vi "Main.vi"(11 "Module Admin":refnum<class "Delacor_lib_QMH_Module Admin.lvclass">) -> ()   [LabVIEW 2020, in "Dinero.lvlib"]
doc: "This template is based off of the Queued Message Handler design pattern and the Queued Message Handler project template that ships with LabVIEW.\n\nThe main difference is that the queue is private to this module and communication between modules is performed via Broadcast and Request events.\n\nRequest events are wrapped in public API methods and are handled in the Event Handling Loop (EHL) of this VI. Any module can register for Broadcast events sent by this module. The EHL generates messages based on user interface actions.\n\nThe Message Handling Loop (MHL) processes messages generated by the EHL, or by other messages. The messages are string values, so new messages can be added easily to the Message Cases case structure in the MHL. Each message cluster can also provide an optional value for Message Data, which is a variant that can be converted to whatever message-specific data is required.\n_____\nBased on DQMH Project Template 6.0.0.91."
uses:
  Dinero.lvlib
  <vilib>/Delacor/Delacor QMH/Libraries/Module Admin_class/Delacor_lib_QMH_Module Admin.lvclass
  Module Data--cluster.ctl
  Stop Argument--cluster.ctl
  <vilib>/Delacor/Delacor QMH/Libraries/Message Queue_class/Delacor_lib_QMH_Message Queue.lvclass/Delacor_lib_QMH_Message Queue.ctl
  <vilib>/Delacor/Delacor QMH/Libraries/Module Admin_class/Delacor_lib_QMH_Module Admin.lvclass/Delacor_lib_QMH_Module Admin.ctl
  DRAW FP IN UI Argument--cluster.ctl
  Moneda 1 Argument--cluster.ctl
  Moneda 2 Argument--cluster.ctl
  Moneda 5 Argument--cluster.ctl
  Moneda 10 Argument--cluster.ctl
  <vilib>/Utility/miscctls.llb/LVPointTypeDef.ctl
  <vilib>/Delacor/Delacor QMH/Libraries/Message Queue_class/Delacor_lib_QMH_Enqueue Message (Single).vi
  <vilib>/Delacor/Delacor QMH/Libraries/Module Admin_class/Delacor_lib_QMH_Get External Launch.vi
  <vilib>/Utility/error.llb/Error Cluster From Error Code.vi
  <vilib>/ErrorRing/Error Ring.xnode
  <vilib>/Delacor/Delacor QMH/Libraries/Message Queue_class/Delacor_lib_QMH_Message Queue.lvclass
panel:
  out "Cambio":i32
  out "Credito":i32
  in  "Moneda 4":bool
  in  "Moneda 3":bool
  in  "Moneda 2":bool
  in  "Moneda 1":bool
  out "error out":errorcluster
  out "Status":string
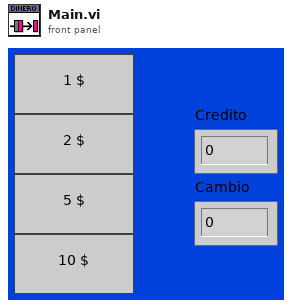
[diagram p1: front panel]
types:
  T1 = typedef "Dinero.lvlib/Request Events--cluster.ctl" = cluster{"Stop Module":refnum<user-event>, "Show Panel":refnum<user-event>, "Hide Panel":refnum<user-event>, "Get Module Execution Status":refnum<user-event>, "Show Diagram":refnum<user-event>, "DRAW FP IN UI":refnum<user-event>, "Moneda 1":refnum<user-event>, "Moneda 2":refnum<user-event>, "Moneda 5":refnum<user-event>, "Moneda 10":refnum<user-event>}
  T2 = typedef "Dinero.lvlib/Module Data--cluster.ctl" = cluster{"Status":string, "Credito":i32, "Cambio":i32}
  T3 = enum32{"invalid lock state", "Not Locked", "Locked (No Password)", "Password-protected"}
  T4 = typedef "Dinero.lvlib/Stop Argument--cluster.ctl" = cluster{"Origin":string, "Exit via Stop Module Req?":bool, "Wait for Module to stop?":bool}
  T5 = typedef "Dinero.lvlib/DRAW FP IN UI Argument--cluster.ctl" = cluster{"Sub Panel Dinero":refnum<vi>}
  T6 = typedef "Dinero.lvlib/Moneda 1 Argument--cluster.ctl" = cluster{"Boolean":bool}
  T7 = typedef "Dinero.lvlib/Moneda 2 Argument--cluster.ctl" = cluster{"Boolean":bool}
  T8 = typedef "Dinero.lvlib/Moneda 5 Argument--cluster.ctl" = cluster{"Boolean":bool}
  T9 = typedef "Dinero.lvlib/Moneda 10 Argument--cluster.ctl" = cluster{"Boolean":bool}
  T10 = typedef "LVPointTypeDef.ctl" = cluster{"Horizontal":i16, "Vertical":i16}
  T11 = enum32{"Invalid", "Standard", "Closed", "Hidden", "Minimized", "Maximized"}
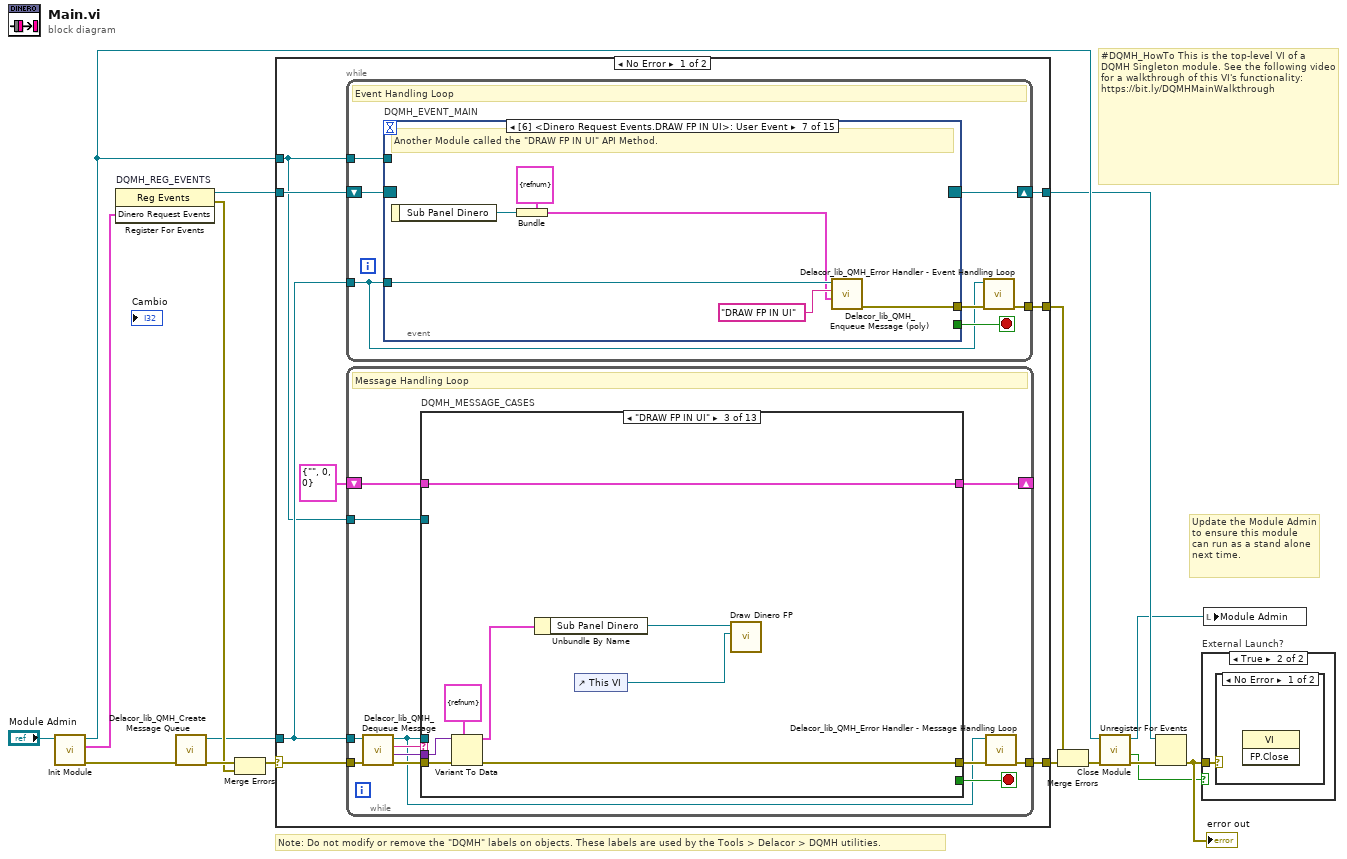
[diagram p0: block diagram]
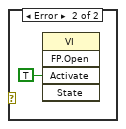
[diagram p3: hidden frame]
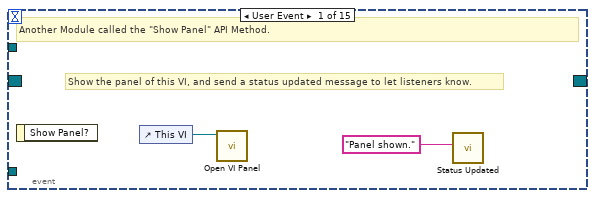
[diagram p4: hidden frame]
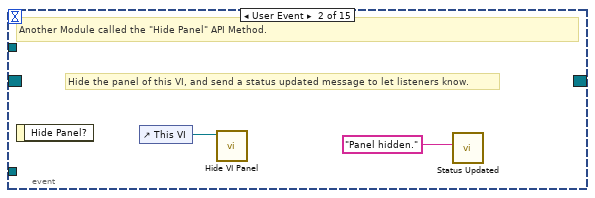
[diagram p5: hidden frame]
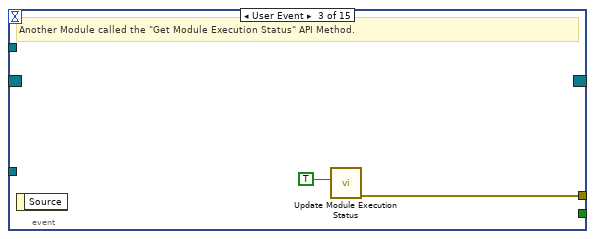
[diagram p6: hidden frame]
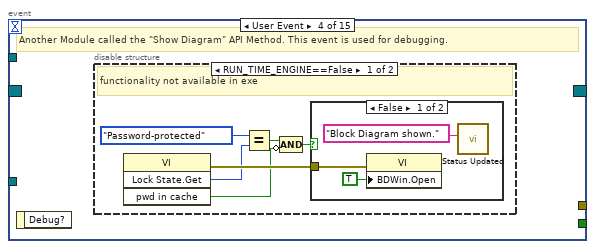
[diagram p7: hidden frame]
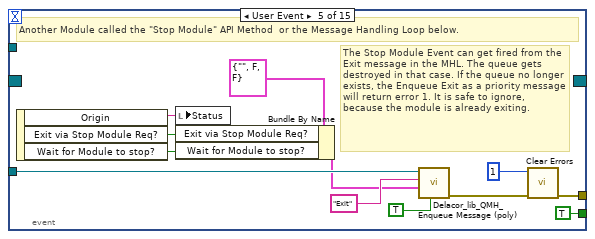
[diagram p10: hidden frame]
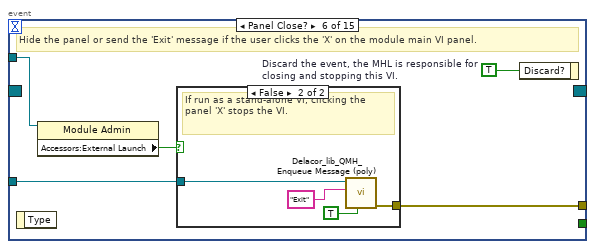
[diagram p11: hidden frame]
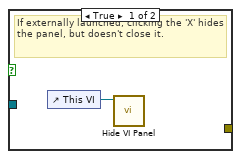
[diagram p12: hidden frame]
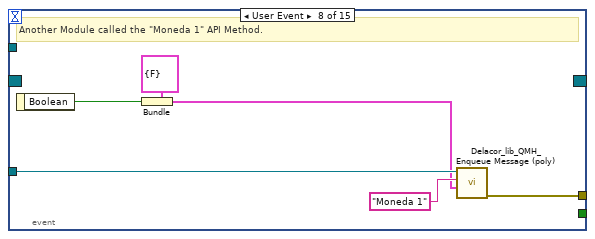
[diagram p13: hidden frame]
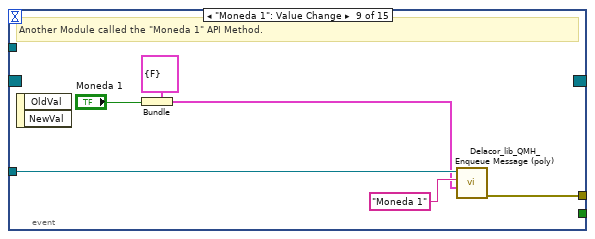
[diagram p14: hidden frame]
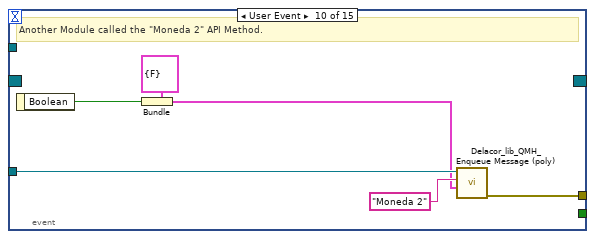
[diagram p15: hidden frame]
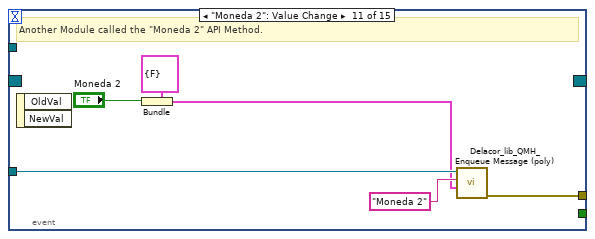
[diagram p16: hidden frame]
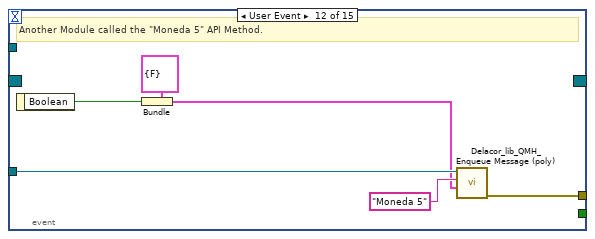
[diagram p17: hidden frame]
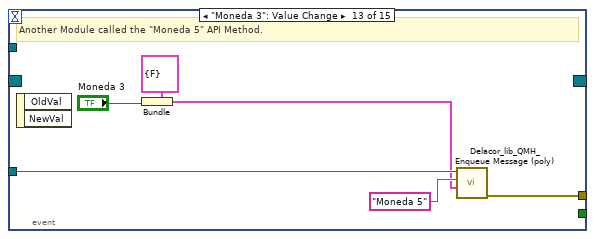
[diagram p18: hidden frame]
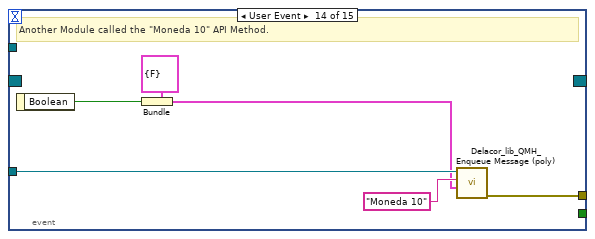
[diagram p19: hidden frame]
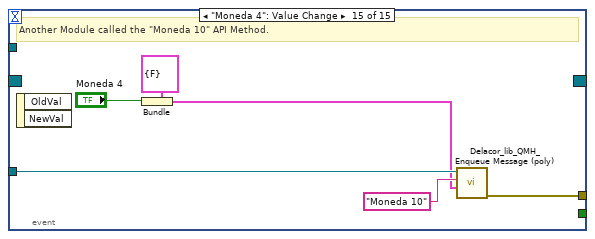
[diagram p20: hidden frame]
diagram:
  # "#DQMH_HowTo This is the top-level VI of a DQMH Singleton module. See the following video for a walkthrough of this VI's functionality: https://bit.ly/DQMHMainWalkthrough"
  # "Note: Do not modify or remove the \"DQMH\" labels on objects. These labels are used by the Tools > Delacor > DQMH utilities."
  # "Update the Module Admin to ensure this module can run as a stand alone next time."
  n1 = call "Init Module.vi"("Singleton Module Admin in"="Module Admin") -> ("error out"=w16:errorcluster, "Dinero Request Events"=w5:T1, "Singleton Module Admin out"=w8:refnum<class "Delacor_lib_QMH_Module Admin.lvclass">)  [unwired: 8 in]
  n2 = register-events "DQMH_REG_EVENTS"(w5) -> (reference out=w6:refnum<event-registration>, error out=w9:errorcluster)  [unwired: 2 in]
  n3 = call <vilib>:"Delacor_lib_QMH_Create Message Queue.vi"("error in"=w16) -> ("error out"=w11:errorcluster, "Message Queue"=w4:refnum<class "Delacor_lib_QMH_Message Queue.lvclass">)  [unwired: 9 in]
  n4 = Merge Errors(w11, w9) -> (w10:errorcluster)
  n5 = case shown="No Error" w10 {
    selector: w10 -> [w23 w273]
    tunnel: [w25 w272] -> w17
    tunnel: [w22 w278] -> w7
    tunnel: w6 -> [w20 w278]
    tunnel: w4 -> [w19 w271]
    tunnel: [w24 _] -> w14
    tunnel: w8 -> [w18 w274]
    frame No Error {
      n6 = while {
        tunnel: w19 -> [w26]
        shift-right: [w29] -> w22
        shift-left: w20 -> [w30]
        tunnel: [w31] -> w24
        tunnel: w18 -> [w27]
        stop <- w28 stop-if-true
        # "Event Handling Loop"
        n7 = event "DQMH_EVENT_MAIN" shown="[6] <Dinero Request Events.DRAW FP IN UI>: User Event" {
          selector: w30 -> [_ _ _ _ _ _ _ _ _ _ _ _ _ _ _]
          dyn-events: [_ _ _ _ _ _ _ _ _ _ _ _ _ _ _] -> w29
          timeout: _ -> [_ _ _ _ _ _ _ _ _ _ _ _ _ _ _]
          tunnel: [_ _ _ _ TRUE ("Discard?") _ _ _ _ _ _ _ _ _ _] -> w28
          tunnel: w26 -> [_ _ _ _ w55 w62 w75 w81 w87 w93 w99 w105 w111 w117 w123]
          tunnel: [_ _ w38 _ w58 w64 w70 w76 w83 w88 w95 w100 w107 w112 w119] -> w32
          tunnel: w27 -> [_ _ _ _ _ w61 _ _ _ _ _ _ _ _ _]
          event User Event {
            # "Show the panel of this VI, and send a status updated message to let listeners know."
            # "Another Module called the \"Show Panel\" API Method."
            n8 = event-data() -> ()  [unwired: 1 in, 1 out]
            n9 = control-ref of="This VI"() -> (w34:refnum<vi>)
            n10 = call "Open VI Panel.vi"("VI"=w34) -> ()  [unwired: 10 in, 1 out]
            n11 = call "Status Updated.vi"("Status"="Panel shown." ("format string")) -> ()  [unwired: 10 in, 1 out]
          }
          event User Event {
            # "Hide the panel of this VI, and send a status updated message to let listeners know."
            # "Another Module called the \"Hide Panel\" API Method."
            n12 = event-data() -> ()  [unwired: 1 in, 1 out]
            n13 = control-ref of="This VI"() -> (w36:refnum<vi>)
            n14 = call "Hide VI Panel.vi"("VI"=w36) -> ()  [unwired: 10 in, 1 out]
            n15 = call "Status Updated.vi"("Status"="Panel hidden." ("format string")) -> ()  [unwired: 10 in, 1 out]
          }
          event User Event {
            # "Another Module called the \"Get Module Execution Status\" API Method."
            n16 = event-data() -> ()  [unwired: 1 in, 1 out]
            n17 = call "Update Module Execution Status.vi"("Running?"=TRUE) -> ("error out"=w38:errorcluster)  [unwired: 10 in]
          }
          event User Event {
            # "Another Module called the \"Show Diagram\" API Method. This event is used for debugging."
            n18 = event-data() -> ()  [unwired: 1 in, 1 out]
            n19 = disable-structure shown="RUN_TIME_ENGINE==False" {
              frame condition #0 (active) {
                # "functionality not available in exe"
                n20 = invoke class="VI" method="Lock State.Get"() -> (error out=w44:errorcluster, "Get Lock State"=w43:T3, "pwd in cache"=w40:bool)  [unwired: 4 in, 1 out]
                n21 = Equal?(x=T3."Password-protected", y=w43) -> (x = y?=w41:bool)
                n22 = Compound Arithmetic op=AND(w41, invert w40) -> (w39:bool)
                n23 = case shown="False" w39 {
                  tunnel: w44 -> [w47 _]
                  frame False {
                    n24 = property class="VI"(error in=w47, "BDWin.Open"=TRUE ("Block Diagram Window:Open")) -> ()  [unwired: 1 in, 2 out]
                    n25 = call "Status Updated.vi"("Status"="Block Diagram shown." ("format string")) -> ()  [unwired: 10 in, 1 out]
                  }
                  frame True {
                    # "Password-protected VI, and the password is not in the cache. Do not show the diagram."
                  }
                }
              }
              frame condition #1 {
              }
            }
          }
          event User Event {
            # "The Stop Module Event can get fired from the Exit message in the MHL. The queue gets destroyed in that case. If the queue no longer exists, the Enqueue Exit as a priority message will return error 1. It is safe to ignore, because the module is already exiting."
            # "Another Module called the \"Stop Module\" API Method  or the Message Handling Loop below."
            n26 = event-data() -> ("Origin"=w54:string, "Exit via Stop Module Req?"=w50:bool, "Wait for Module to stop?"=w49:bool)  [unwired: 1 in]
            n27 = local write "Status"(w54) -> ()
            n28 = Bundle By Name(cluster=T4 {"Origin"="", "Exit via Stop Module Req?"=FALSE, "Wait for Module to stop?"=FALSE} ("Stop Argument"), "Exit via Stop Module Req?"=w50, "Wait for Module to stop?"=w49) -> (w48:T4)
            n29 = call-poly <vilib>:"Delacor_lib_QMH_Enqueue Message (poly).vi"("Priority Message? (F)"=TRUE, "Message Data"=w48, "Message"="Exit", "Message Queue in"=w55) -> ("error out"=w59:errorcluster)  [unwired: 6 in, 1 out]
            n30 = call <vilib>:"Clear Errors.vi"("error in (no error)"=w59, "specific error code to clear (0: all)"=1) -> ("error out"=w58:errorcluster)  [unwired: 4 in, 1 out]
          }
          event Panel Close? {
            w63 = TRUE  # Discard the event, the MHL is responsible for closing and stopping this VI.
            # "Hide the panel or send the 'Exit' message if the user clicks the 'X' on the module main VI panel."
            n31 = event-data() -> ()  [unwired: 1 in, 1 out]
            n32 = property class="Module Admin"(reference=w61) -> ("Accessors:External Launch"=w60:bool)  [unwired: 1 in, 2 out]
            n33 = case shown="False" w60 {
              tunnel: w62 -> [_ w68]
              tunnel: [_ w69] -> w64
              frame True {
                # "If externally launched, clicking the 'X' hides the panel, but doesn't close it."
                n34 = control-ref of="This VI"() -> (w65:refnum<vi>)
                n35 = call "Hide VI Panel.vi"("VI"=w65) -> ()  [unwired: 10 in, 1 out]
              }
              frame False {
                # "If run as a stand-alone VI, clicking the panel 'X' stops the VI."
                n36 = call-poly <vilib>:"Delacor_lib_QMH_Enqueue Message (poly).vi"("Priority Message? (F)"=TRUE, "Message"="Exit", "Message Queue in"=w68) -> ("error out"=w69:errorcluster)  [unwired: 7 in, 1 out]
              }
            }
            n37 = event-data("Discard?"=w63) -> ()  [unwired: 1 in, 1 out]
          }
          event User Event {
            # "Another Module called the \"DRAW FP IN UI\" API Method."
            n38 = event-data() -> ("Sub Panel Dinero"=w71:refnum<vi>)  [unwired: 1 in]
            n39 = Bundle(cluster=T5 {"Sub Panel Dinero"=refnum} ("DRAW FP IN UI Argument"), "Sub Panel Dinero"=w71) -> (w72:T5)
            n40 = call-poly <vilib>:"Delacor_lib_QMH_Enqueue Message (poly).vi"("Message Data"=w72, "Message"="DRAW FP IN UI", "Message Queue in"=w75) -> ("error out"=w70:errorcluster)  [unwired: 7 in, 1 out]
          }
          event User Event {
            # "Another Module called the \"Moneda 1\" API Method."
            n41 = event-data() -> ("Boolean"=w77:bool)  [unwired: 1 in]
            n42 = Bundle(cluster=T6 {"Boolean"=FALSE} ("Moneda 1 Argument"), "Boolean"=w77) -> (w78:T6)
            n43 = call-poly <vilib>:"Delacor_lib_QMH_Enqueue Message (poly).vi"("Message Data"=w78, "Message"="Moneda 1", "Message Queue in"=w81) -> ("error out"=w76:errorcluster)  [unwired: 7 in, 1 out]
          }
          event "Moneda 1": Value Change {
            # "Another Module called the \"Moneda 1\" API Method."
            n44 = event-data() -> ()  [unwired: 1 in, 2 out]
            n45 = Bundle(cluster=T6 {"Boolean"=FALSE} ("Moneda 1 Argument"), "Boolean"="Moneda 1") -> (w84:T6)
            n46 = call-poly <vilib>:"Delacor_lib_QMH_Enqueue Message (poly).vi"("Message Data"=w84, "Message"="Moneda 1", "Message Queue in"=w87) -> ("error out"=w83:errorcluster)  [unwired: 7 in, 1 out]
          }
          event User Event {
            # "Another Module called the \"Moneda 2\" API Method."
            n47 = event-data() -> ("Boolean"=w89:bool)  [unwired: 1 in]
            n48 = Bundle(cluster=T7 {"Boolean"=FALSE} ("Moneda 2 Argument"), "Boolean"=w89) -> (w90:T7)
            n49 = call-poly <vilib>:"Delacor_lib_QMH_Enqueue Message (poly).vi"("Message Data"=w90, "Message"="Moneda 2", "Message Queue in"=w93) -> ("error out"=w88:errorcluster)  [unwired: 7 in, 1 out]
          }
          event "Moneda 2": Value Change {
            # "Another Module called the \"Moneda 2\" API Method."
            n50 = event-data() -> ()  [unwired: 1 in, 2 out]
            n51 = Bundle(cluster=T7 {"Boolean"=FALSE} ("Moneda 2 Argument"), "Boolean"="Moneda 2") -> (w96:T7)
            n52 = call-poly <vilib>:"Delacor_lib_QMH_Enqueue Message (poly).vi"("Message Data"=w96, "Message"="Moneda 2", "Message Queue in"=w99) -> ("error out"=w95:errorcluster)  [unwired: 7 in, 1 out]
          }
          event User Event {
            # "Another Module called the \"Moneda 5\" API Method."
            n53 = event-data() -> ("Boolean"=w101:bool)  [unwired: 1 in]
            n54 = Bundle(cluster=T8 {"Boolean"=FALSE} ("Moneda 5 Argument"), "Boolean"=w101) -> (w102:T8)
            n55 = call-poly <vilib>:"Delacor_lib_QMH_Enqueue Message (poly).vi"("Message Data"=w102, "Message"="Moneda 5", "Message Queue in"=w105) -> ("error out"=w100:errorcluster)  [unwired: 7 in, 1 out]
          }
          event "Moneda 3": Value Change {
            # "Another Module called the \"Moneda 5\" API Method."
            n56 = event-data() -> ()  [unwired: 1 in, 2 out]
            n57 = Bundle(cluster=T8 {"Boolean"=FALSE} ("Moneda 5 Argument"), "Boolean"="Moneda 3") -> (w108:T8)
            n58 = call-poly <vilib>:"Delacor_lib_QMH_Enqueue Message (poly).vi"("Message Data"=w108, "Message"="Moneda 5", "Message Queue in"=w111) -> ("error out"=w107:errorcluster)  [unwired: 7 in, 1 out]
          }
          event User Event {
            # "Another Module called the \"Moneda 10\" API Method."
            n59 = event-data() -> ("Boolean"=w113:bool)  [unwired: 1 in]
            n60 = Bundle(cluster=T9 {"Boolean"=FALSE} ("Moneda 10 Argument"), "Boolean"=w113) -> (w114:T9)
            n61 = call-poly <vilib>:"Delacor_lib_QMH_Enqueue Message (poly).vi"("Message Data"=w114, "Message"="Moneda 10", "Message Queue in"=w117) -> ("error out"=w112:errorcluster)  [unwired: 7 in, 1 out]
          }
          event "Moneda 4": Value Change {
            # "Another Module called the \"Moneda 10\" API Method."
            n62 = event-data() -> ()  [unwired: 1 in, 2 out]
            n63 = Bundle(cluster=T9 {"Boolean"=FALSE} ("Moneda 10 Argument"), "Boolean"="Moneda 4") -> (w120:T9)
            n64 = call-poly <vilib>:"Delacor_lib_QMH_Enqueue Message (poly).vi"("Message Data"=w120, "Message"="Moneda 10", "Message Queue in"=w123) -> ("error out"=w119:errorcluster)  [unwired: 7 in, 1 out]
          }
        }
        n65 = call-dynamic "Delacor_lib_QMH_Error Handler - Event Handling Loop.vi"("error in"=w32, "Message Queue in"=w26) -> ("dup error in"=w31:errorcluster)  [unwired: 8 in, 1 out]
      }
      n66 = while {
        tunnel: w19 -> [w126]
        shift-right: [w130] -> _
        shift-left: T2 {"Status"="", "Credito"=0, "Cambio"=0} ("Data Cluster") -> [w131]
        tunnel: w23 -> [w134]
        tunnel: [w132] -> w25
        tunnel: w18 -> [w124]
        stop <- w129 stop-if-true
        # "Message Handling Loop"
        n67 = call-dynamic "Delacor_lib_QMH_Dequeue Message.vi"("error in"=w134, "Message Queue in"=w126) -> ("error out"=w133:errorcluster, "Message Data"=w127:variant, "Message"=w128:string, "Message Queue out"=w125:refnum<class "Delacor_lib_QMH_Message Queue.lvclass">)  [unwired: 6 in]
        n68 = case "DQMH_MESSAGE_CASES" shown="\"DRAW FP IN UI\"" w128 {
          selector: w128 -> [_ _ _ _ _ _ _ _ _ _ _ _ w258]
          tunnel: w125 -> [_ _ _ w168 w179 w192 w206 _ _ _ w228 w250 _]
          tunnel: w133 -> [w153 w157 w165 w178 w191 w204 w217 w220 w223 w225 w235 w256 w260]
          tunnel: [w151 w157 w163 w166 w180 w193 w207 w220 w222 w225 w231 w253 w261] -> w135
          tunnel: w131 -> [w142 w156 w164 w174 w184 w197 w210 w219 w221 w224 w230 w249 w259]
          tunnel: [w141 w156 w164 w173 w183 w196 w209 w219 w221 w224 w230 w249 w259] -> w130
          tunnel: [_ _ _ _ _ _ _ _ _ _ _ w248 _] -> w129
          tunnel: w127 -> [_ _ w162 w177 w190 w203 w216 _ _ _ w229 w247 _]
          tunnel: w124 -> [w143 _ _ _ _ _ _ _ _ _ w227 w242 _]
          frame "Initialize" {
            w137 = "Initial Message" ("Initial Message")
            # "Initialize - Any operation that needs to be done before the module can receive messages. Synchronize Caller Events.vi will inform Start Module.vi that the module has launched and is ready to receive messages. Module Did Init.vi will broadcast that the module initialized."
            n69 = call "Synchronize Caller Events.vi"("error in (no error)"=w153, "Singleton Module Admin in"=w143) -> ("error out"=w152:errorcluster, "Singleton Module Admin out"=w138:refnum<class "Delacor_lib_QMH_Module Admin.lvclass">)  [unwired: 8 in]
            n70 = property class="Module Admin"(reference=w138) -> ("Accessors:External Launch"=w147:bool)  [unwired: 1 in, 2 out]
            n71 = Select(t=T11."Hidden" ("State"), s=w147, f=T11."Standard" ("State")) -> (s? t:f=w144:T11)
            n72 = call "Module Name--constant.vi"() -> ("Module Name"=w150:string)  [unwired: 11 in]
            n73 = property class="VI"("Front Panel.Title"=w150) -> (reference out=w149:refnum<vi>, error out=w155:errorcluster)  [unwired: 2 in]
            n74 = call "Module Name--constant.vi"() -> ("Module Name"=w139:string)  [unwired: 11 in]
            n75 = invoke class="VI" method="FP.Open"(reference=w149, error in=w155, "State"=w144) -> (reference out=w148:refnum<vi>, error out=w154:errorcluster)  [unwired: 2 in, 3 out]
            n76 = Bundle By Name(cluster=w142, "Status"=w137) -> (w141:T2)
            n77 = call "Module Did Init.vi"("error in (no error)"=w152, "Initialized?"=TRUE, "Origin"=w139) -> ("error out"=w151:errorcluster)  [unwired: 8 in]
            n78 = invoke class="VI" method="FP.Center"(reference=w148, error in=w154) -> ()  [unwired: 1 in, 3 out]
            n79 = property on="Pane" class="Pane"("Origin"=T10 {"Horizontal"=0, "Vertical"=0}) -> ()  [unwired: 2 in, 2 out]
            "Status" <- w137
          }
          frame "---Module Specific---" {
            # "Separator -- The following cases handle messages specific to this Module."
          }
          frame "DRAW FP IN UI" {
            n80 = Variant To Data(error in=w165, type=T5 {"Sub Panel Dinero"=refnum} ("DRAW FP IN UI Argument"), Variant=w162) -> (data=w160:T5, error out=w163:errorcluster)
            n81 = Unbundle By Name(w160) -> ("Sub Panel Dinero"=w159:refnum<vi>)
            n82 = control-ref of="This VI"() -> (w158:refnum<vi>)
            n83 = call "Draw Dinero FP.vi"("This VI Dinero"=w158, "Sub Panel Dinero"=w159) -> ()  [unwired: 10 in]
          }
          frame "Moneda 1" {
            n84 = Variant To Data(error in=w178, type=T6 {"Boolean"=FALSE} ("Moneda 1 Argument"), Variant=w177) -> (data=w175:T6, error out=w167:errorcluster)
            n85 = Unbundle By Name(w174) -> ("Credito"=w172:i32)
            n86 = Unbundle By Name(w175) -> ()  [unwired: 1 out]
            n87 = call "Select Moneda.vi"("Moneda"=1, "Credito"=w172) -> ("New Credit"=w170:i32)  [unwired: 9 in]
            n88 = call-poly <vilib>:"Delacor_lib_QMH_Enqueue Message (poly).vi"("error in"=w167, "Message"="Update Credito", "Message Queue in"=w168) -> ("error out"=w166:errorcluster)  [unwired: 7 in, 1 out]
            n89 = Bundle By Name(cluster=w174, "Credito"=w170) -> (w173:T2)
          }
          frame "Moneda 2" {
            n90 = Variant To Data(error in=w191, type=T7 {"Boolean"=FALSE} ("Moneda 2 Argument"), Variant=w190) -> (data=w188:T7, error out=w181:errorcluster)
            n91 = Unbundle By Name(w184) -> ("Credito"=w187:i32)
            n92 = Unbundle By Name(w188) -> ()  [unwired: 1 out]
            n93 = call "Select Moneda.vi"("Moneda"=2, "Credito"=w187) -> ("New Credit"=w185:i32)  [unwired: 9 in]
            n94 = Bundle By Name(cluster=w184, "Credito"=w185) -> (w183:T2)
            n95 = call-poly <vilib>:"Delacor_lib_QMH_Enqueue Message (poly).vi"("error in"=w181, "Message"="Update Credito", "Message Queue in"=w179) -> ("error out"=w180:errorcluster)  [unwired: 7 in, 1 out]
          }
          frame "Moneda 5" {
            n96 = Variant To Data(error in=w204, type=T8 {"Boolean"=FALSE} ("Moneda 5 Argument"), Variant=w203) -> (data=w201:T8, error out=w194:errorcluster)
            n97 = Unbundle By Name(w197) -> ("Credito"=w200:i32)
            n98 = Unbundle By Name(w201) -> ()  [unwired: 1 out]
            n99 = call "Select Moneda.vi"("Moneda"=5, "Credito"=w200) -> ("New Credit"=w198:i32)  [unwired: 9 in]
            n100 = Bundle By Name(cluster=w197, "Credito"=w198) -> (w196:T2)
            n101 = call-poly <vilib>:"Delacor_lib_QMH_Enqueue Message (poly).vi"("error in"=w194, "Message"="Update Credito", "Message Queue in"=w192) -> ("error out"=w193:errorcluster)  [unwired: 7 in, 1 out]
          }
          frame "Moneda 10" {
            n102 = Variant To Data(error in=w217, type=T9 {"Boolean"=FALSE} ("Moneda 10 Argument"), Variant=w216) -> (data=w214:T9, error out=w208:errorcluster)
            n103 = Unbundle By Name(w210) -> ("Credito"=w213:i32)
            n104 = Unbundle By Name(w214) -> ()  [unwired: 1 out]
            n105 = call "Select Moneda.vi"("Moneda"=10, "Credito"=w213) -> ("New Credit"=w211:i32)  [unwired: 9 in]
            n106 = call-poly <vilib>:"Delacor_lib_QMH_Enqueue Message (poly).vi"("error in"=w208, "Message"="Update Credito", "Message Queue in"=w206) -> ("error out"=w207:errorcluster)  [unwired: 7 in, 1 out]
            n107 = Bundle By Name(cluster=w210, "Credito"=w211) -> (w209:T2)
          }
          frame "Update Credito" {
            n108 = Unbundle By Name(w219) -> ("Credito"=→"Credito":i32)
          }
          frame "---Copy This Frame---" {
            # "Duplicate this frame when creating new messages.  Change this comment in the duplicated frame to describe this message."
            n109 = Merge Errors(w223) -> (w222:errorcluster)
          }
          frame "---Exit and Error Handling---" {
            # "Separator - The following cases handle errors and exit messages."
          }
          frame "Error" {
            # "#CodeRecommended - If you ever change the name of this \"Error\" message, you'll need to update the name in the Check Loop Error.vi as well."
            # "#CodeRecommended - If the module is running in standalone mode (External Launch = FALSE), this code will pop up an error dialog and call the 'Exit' message if an error occurs. Add more fine-grained error handling here."
            # "Error - Check the error message data and respond accordingly. This message is sent by the \"Error Handler\" VIs at the end of each loop in this application."
            n110 = property class="Module Admin"(reference=w227) -> ("Accessors:External Launch"=w226:bool)  [unwired: 1 in, 2 out]
            n111 = Variant To Data(error in=w235, type=errorcluster {"status"=FALSE, "code"=0, "source"=""} ("error constant"), Variant=w229) -> (data=w236:errorcluster, error out=w233:errorcluster)
            n112 = call "Error Reported.vi"("Error"=w236) -> ()  [unwired: 10 in, 1 out]
            n113 = case shown="False" w226 {
              tunnel: [w241 _] -> w232
              tunnel: w228 -> [w239 _]
              tunnel: w236 -> [w240 _]
              frame False {
                # "If the module is running standalone, then pop up an error dialog and call the \"Exit\" message."
                n114 = call <vilib>:"Simple Error Handler.vi"("error in (no error)"=w240) -> ()  [unwired: 4 in, 5 out]
                n115 = call-poly <vilib>:"Delacor_lib_QMH_Enqueue Message (poly).vi"("Priority Message? (F)"=TRUE, "Message"="Exit", "Message Queue in"=w239) -> ("error out"=w241:errorcluster)  [unwired: 7 in, 1 out]
              }
              frame True {
                # "If the module was launched externally, calling the Error Reported broadcast VI is the only action performed by the \"Error\" message. The module's caller can then process the error appropriately."
              }
            }
            n116 = Merge Errors(w233, w232) -> (w231:errorcluster)
            n117 = local write "error out"(w231) -> ()
          }
          frame "Exit" {
            w246 = 91  # 91: not all Exit messages will have an argument
            w248 = TRUE  # Stop the VI
            # "Release the message queue reference"
            # "#CodeNeeded - Add any required cleanup code here"
            # "Exit - Exit the application."
            n118 = Variant To Data(error in=w256, type=T4 {"Origin"="", "Exit via Stop Module Req?"=FALSE, "Wait for Module to stop?"=FALSE} ("Stop Argument"), Variant=w247) -> (data=w244:T4, error out=w252:errorcluster)
            n119 = call <vilib>:"Clear Errors.vi"("error in (no error)"=w252, "specific error code to clear (0: all)"=w246) -> ("error out"=w255:errorcluster)  [unwired: 4 in, 1 out]
            n120 = control-ref of="This VI"() -> (w243:refnum<vi>)
            n121 = call-dynamic "Delacor_lib_QMH_Release Message Queue.vi"("error in"=w255, "Message Queue"=w250) -> ("error out"=w254:errorcluster)  [unwired: 9 in]
            n122 = call "Handle Exit.vi"("Stop Argument"=w244, "Admin in"=w242, "VI reference"=w243) -> ("error out"=w251:errorcluster)  [unwired: 7 in, 1 out]
            n123 = Merge Errors(w254, w251) -> (w253:errorcluster)
          }
          frame Default {
            # "'Default' case only runs if there is a message that isn't defined in any of the other cases.  Output a programming error."
            n124 = call "Module Name--constant.vi"() -> ("Module Name"=w257:string)  [unwired: 11 in]
            n125 = xnode "Error Ring"("parameter 0"=w258, "parameter 1"=w257) -> ("error out"=w262:errorcluster)
            n126 = Merge Errors(w260, w262) -> (w261:errorcluster)
          }
        }
        n127 = call-dynamic "Delacor_lib_QMH_Error Handler - Message Handling Loop.vi"("error in"=w135, "Message Queue in"=w125) -> ("dup error in"=w132:errorcluster)  [unwired: 8 in, 1 out]
      }
    }
    frame Error {
      # "Synchronize Caller Events.vi will inform Start Module.vi that the module has launched and will let the code calling Start Module.vi register for broadcasts and would permit the caller receive the broadcast that an error occurred at launch time."
      n128 = call-dynamic "Delacor_lib_QMH_Release Message Queue.vi"("error in"=w273, "Message Queue"=w271) -> ("error out"=w272:errorcluster)  [unwired: 9 in]
      n129 = call "Synchronize Caller Events.vi"("Singleton Module Admin in"=w274) -> ("error out"=w279:errorcluster)  [unwired: 9 in, 1 out]
      n130 = call "Module Name--constant.vi"() -> ("Module Name"=w277:string)  [unwired: 11 in]
      n131 = Format Into String(format string="An error occurred during initialization. %s is no longer running.", w277) -> (resulting string=w275:string)  [unwired: 2 in, 1 out]
      n132 = Merge Errors(w272, w279) -> (w280:errorcluster)
      n133 = call "Error Reported.vi"("Additional Information"=w275, "Error"=w280) -> ()  [unwired: 9 in, 1 out]
    }
  }
  n134 = Merge Errors(w14, w17) -> (w13:errorcluster)
  n135 = call "Close Module.vi"("error in (no error)"=w13, "Module Admin in"=w8) -> ("error out"=w15:errorcluster, "External Launch"=w1:bool, "Module Admin out"=w2:refnum<class "Delacor_lib_QMH_Module Admin.lvclass">)  [unwired: 7 in]
  n136 = Unregister For Events(event registration refnum=w7, error in=w15) -> (error out=w12:errorcluster)
  "error out" <- w12
  n137 = case "External Launch?" shown="True" w1 {
    tunnel: w12 -> [_ w281]
    frame False {
    }
    frame True {
      n138 = case shown="No Error" w281 {
        frame No Error {
          n139 = invoke class="VI" method="FP.Close"() -> ()  [unwired: 3 in, 3 out]
        }
        frame Error {
          n140 = invoke class="VI" method="FP.Open"("Activate"=TRUE ("Activate?")) -> ()  [unwired: 4 in, 5 out]
        }
      }
    }
  }
  n141 = local write "Module Admin"(w2) -> ()
